vi "getArrayElementByName(recursive).vi"(8 "error in (no error)":errorcluster, 10 "Variant":variant, 11 "ElementHierarchy in":string[](array[string])) -> (0 "error out":errorcluster, 2 "VElement":variant, 3 "ElementOutHierarchy":string[](array[string]))   [LabVIEW 2013]
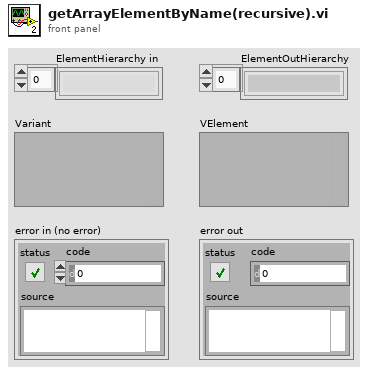
[diagram p1: front panel]
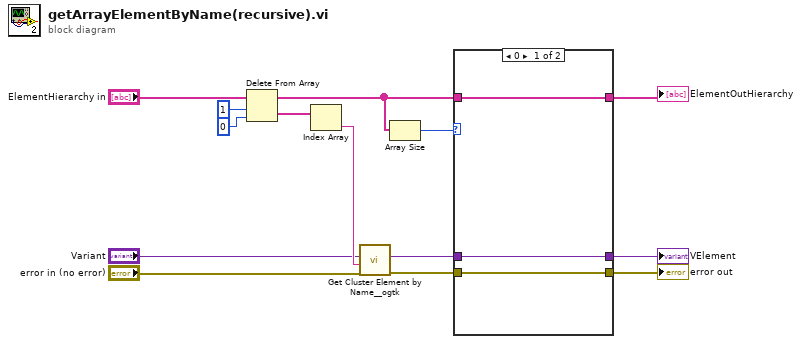
[diagram p0: block diagram]
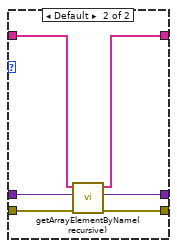
[diagram p2: hidden frame]
diagram:
  n1 = Delete From Array(array="ElementHierarchy in", length=1, index=0) -> (deleted portion=w12:string[], array with subset deleted=w2:string[])
  n2 = Index Array(array=w12) -> (element=w13:string)  [unwired: 1 in]
  n3 = call <userlib>:"Get Cluster Element by Name__ogtk.vi"("error in (no error)"="error in (no error)", "Element Name"=w13, "Cluster"="Variant") -> ("error out"=w4:errorcluster, "VElement"=w6:variant)  [unwired: 6 in, 1 out]
  n4 = Array Size(array=w2) -> (size(s)=w1:i32)
  n5 = case shown="0" w1 {
    tunnel: w2 -> [w17 w23]
    tunnel: [w17 w22] -> w7
    tunnel: w6 -> [w16 w21]
    tunnel: [w16 w20] -> w5
    tunnel: w4 -> [w15 w19]
    tunnel: [w15 w18] -> w3
    frame 0 {
    }
    frame Default {
      n6 = call "getArrayElementByName(recursive).vi"("error in (no error)"=w19, "Variant"=w21, "ElementHierarchy in"=w23) -> ("error out"=w18:errorcluster, "VElement"=w20:variant, "ElementOutHierarchy"=w22:string[])  [unwired: 6 in]
    }
  }
  "ElementOutHierarchy" <- w7
  "VElement" <- w5
  "error out" <- w3
